vi "ExecuteCommand.vi"(11 "Command":string) -> ()   [LabVIEW 2011]
uses:
  <vilib>/Rock Robotics/WPI/DriverStation/DriverStationLCD/WPI_DriverStationLCDLCDLine.ctl
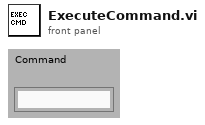
[diagram p1: front panel]
types:
  T1 = typedef "WPI_DriverStationLCDLCDLine.ctl" = enum16{"Main - Line 1", "User - Line 2", "User - Line 3", "User - Line 4", "User - Line 5", "User - Line 6"}
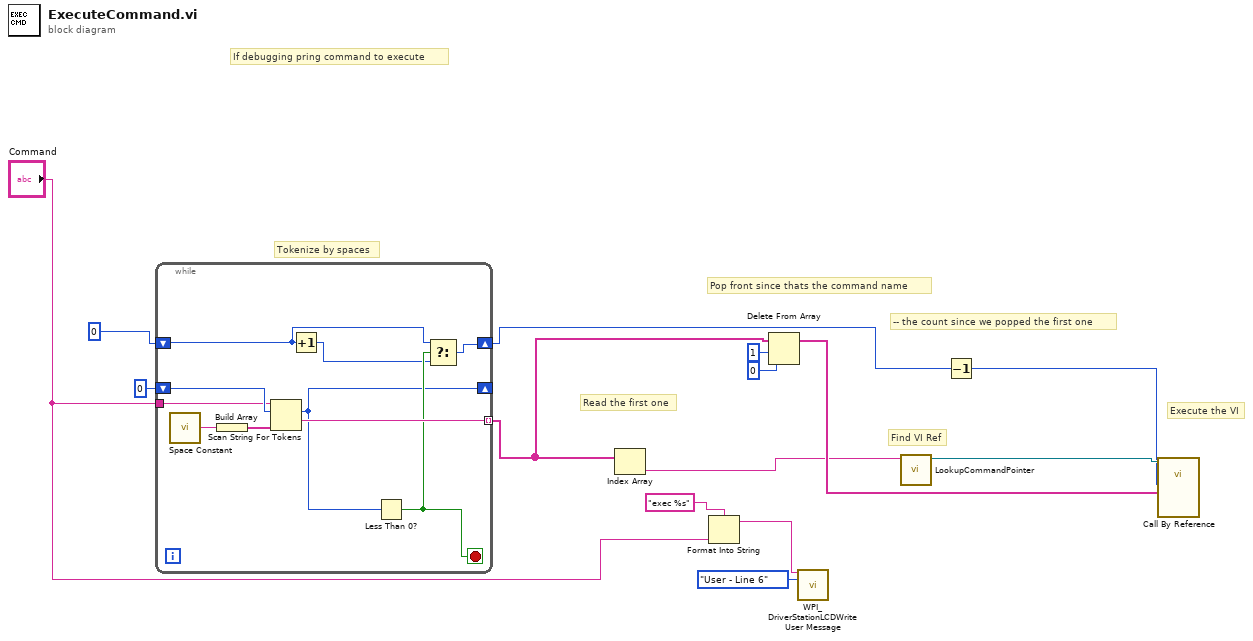
[diagram p0: block diagram]
diagram:
  # "If debugging pring command to execute"
  # "Execute the VI"
  # "-- the count since we popped the first one"
  # "Pop front since thats the command name"
  # "Find VI Ref"
  # "Read the first one"
  # "Tokenize by spaces"
  n1 = while {
    shift-right: [w15] -> _
    shift-left: 0 ("offset past token") -> [w24]
    tunnel: "Command" -> [w23]
    tunnel: [w22] -> w7 mode=indexing
    shift-right: [w18] -> w11
    shift-left: u8 0 -> [w20]
    stop <- w21 stop-if-true
    n2 = call <vilib>:"Space Constant.vi"() -> ("String"=w17:string)
    n3 = Build Array(w17) -> (w16:string[])
    n4 = Scan String For Tokens(6:w16, 8:w24, 9:w23) -> (1:w22:string, 2:w15:i32)  [unwired: 5 out]
    n5 = Increment(x=w20) -> (x+1=w19:u8)
    n6 = Less Than 0?(x=w15) -> (x < 0?=w21:bool)
    n7 = Select(t=w20, s=w21, f=w19) -> (s? t:f=w18:u8)
  }
  n8 = Index Array(array=w7) -> (element=w2:string)  [unwired: 1 in]
  n9 = Format Into String(format string="exec %s" ("initial string"), "Command") -> (resulting string=w3:string)  [unwired: 2 in, 1 out]
  n10 = Delete From Array(array=w7, length=1, index=0) -> (array with subset deleted=w8:string[])  [unwired: 1 out]
  n11 = call <vilib>:"WPI_DriverStationLCDWrite User Message.vi"("line text"=w3, "line"=WPI_DriverStationLCDLCDLine."User - Line 6") -> ()  [unwired: 13 in, 1 out]
  n12 = call "LookupCommandPointer.vi"("refnum name"=w2) -> ("VI Refnum Out"=w10:refnum<vi>)  [unwired: 10 out]
  n13 = Decrement(x=w11) -> (x-1=w9:u8)
  n14 = call-by-ref "?"(reference=w10, "argv"=w8, "args"=w9) -> ()  [unwired: 11 in, 2 out]
